vi "PrepareHWI.vi"(8 "error in (no error)":errorcluster, 9 "Master Device in":refnum<class "Master Device.lvclass">, 10 "Current Variables":T1[](array[typedef]), 11 "Arduino in":refnum<class "Arduino.lvclass">) -> (0 "error out":errorcluster, 2 "Master Device out":refnum<class "Master Device.lvclass">, 3 "Arduino out":refnum<class "Arduino.lvclass">)   [LabVIEW 2013, in "Arduino.lvclass"]
doc: "Prepare HWI will parse string table values to generate a hardware image for each device. Both variables and user functions can be pre-registered! This makes setting variables optional."
uses:
  Arduino.lvclass
  TypeDefs/Active procedure variables.ctl
  Master Device/Master Device.lvclass
  Arduino.lvclass/Arduino.ctl
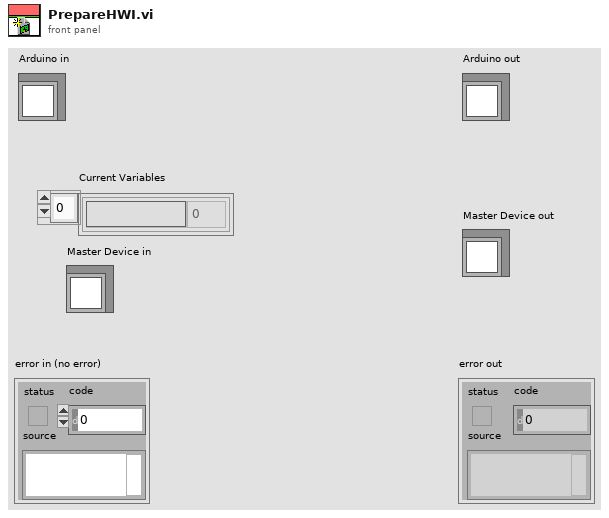
[diagram p1: front panel]
types:
  T1 = typedef "Active procedure variables.ctl" = cluster{"Procedure variable":string, "Value":dbl}
  T2 = cluster{"Short Command":string, "ParamTotal":dbl, "Params":dbl[]}[][]
  T3 = cluster{"Short Command":string, "ParamTotal":dbl, "Params":dbl[]}[]
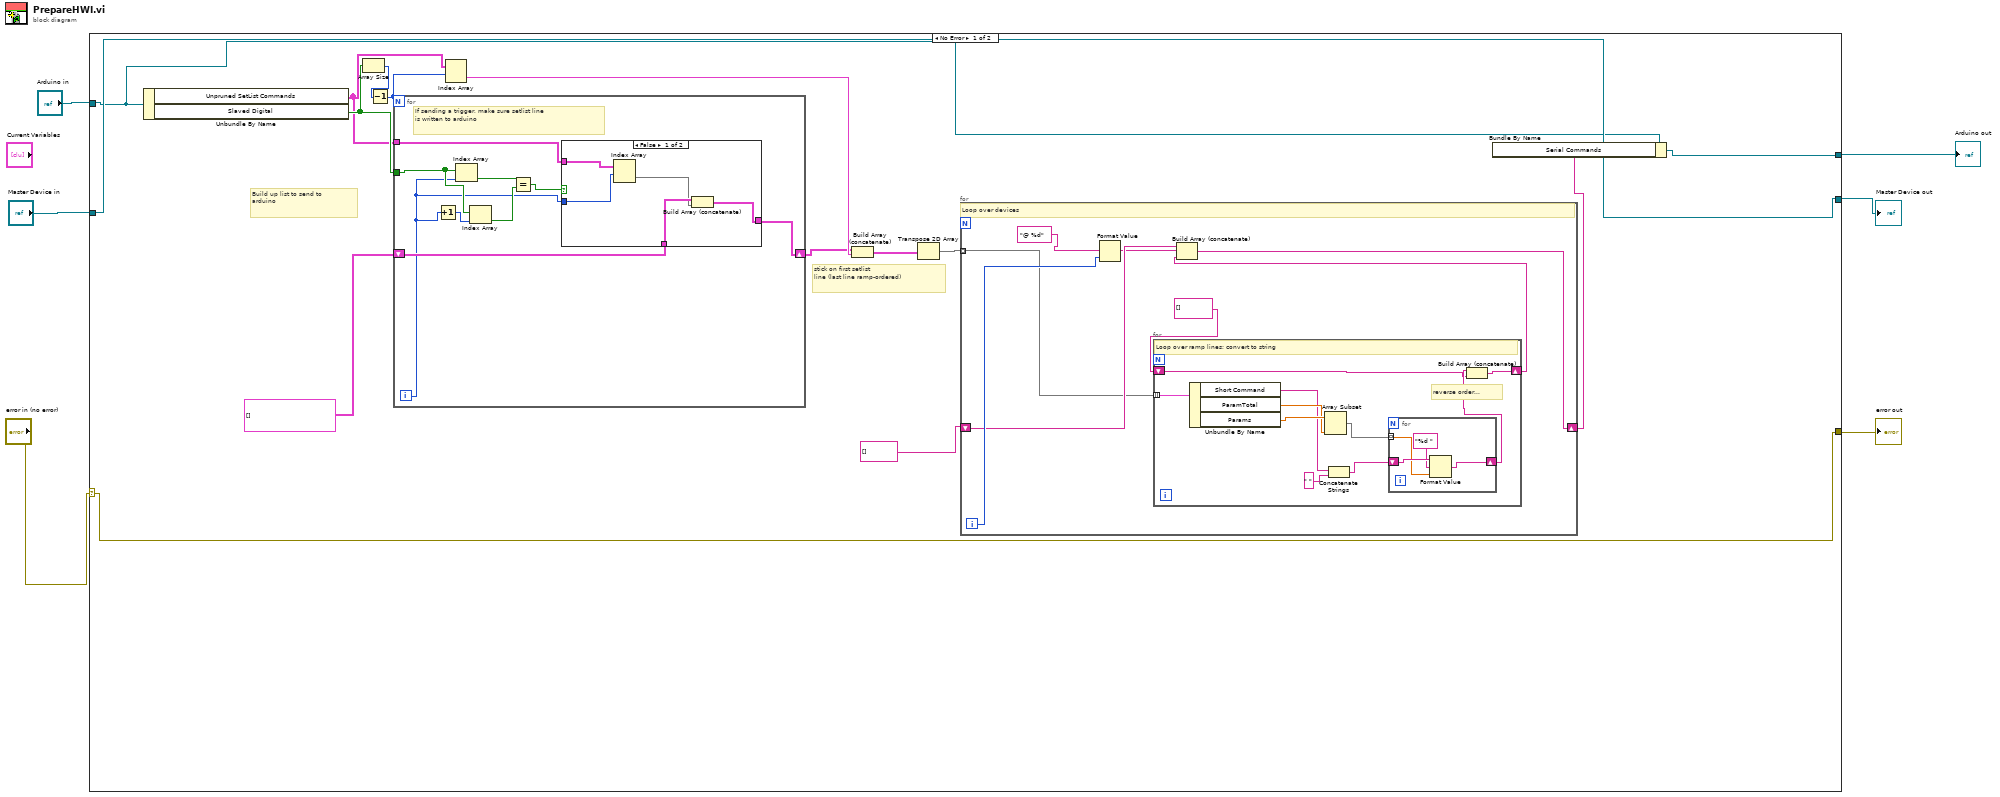
[diagram p0: block diagram]
diagram:
  n1 = case shown="No Error" "error in (no error)" {
    selector: "error in (no error)" -> [w13 w61]
    tunnel: [w13 w61] -> w6
    tunnel: [w19 w60] -> w5
    tunnel: "Master Device in" -> [w19 w60]
    tunnel: [w14 w59] -> w3
    tunnel: "Arduino in" -> [w16 w59]
    frame No Error {
      # "stick on first setlist\nline (last line ramp-ordered)"
      # "Build up list to send to\narduino"
      n2 = Unbundle By Name(w16) -> ("Unpruned SetList Commands"=w11:T2, "Slaved Digital"=w20:bool[])
      n3 = Array Size(array=w20) -> (size(s)=w12:i32)
      n4 = Decrement(x=w12) -> (x-1=w10:i32)
      n5 = for {
        N: w10 -> [_]
        tunnel: w11 -> [w45]
        tunnel: w20 -> [w51]
        shift-right: [w47] -> w8
        shift-left: T2 [] ("Unpruned SetList Commands") -> [w46]
        i -> [w44]
        # "If sending a trigger, make sure setlist line\nis written to arduino"
        n6 = Increment(x=w44) -> (x+1=w52:i32)
        n7 = Index Array(array=w51, index=w44) -> (element=w50:bool)
        n8 = Index Array(array=w51, index=w52) -> (element=w49:bool)
        n9 = Equal?(x=w50, y=w49) -> (x = y?=w48:bool)
        n10 = case shown="False" w48 {
          tunnel: [w56 w58] -> w47
          tunnel: w46 -> [w57 w58]
          tunnel: w45 -> [w55 _]
          tunnel: w44 -> [w54 _]
          frame False {
            n11 = Index Array(array=w55, index (row)=w54) -> (element=w53:T3)  [unwired: 1 in]
            n12 = Build Array (concatenate)(w57, w53) -> (w56:T2)
          }
          frame True {
          }
        }
      }
      n13 = Index Array(array=w11, index (row)=w10) -> (element=w9:T3)  [unwired: 1 in]
      n14 = Build Array (concatenate)(w8, w9) -> (w7:T2)
      n15 = Transpose 2D Array(2D array=w7) -> (transposed array=w18:T2)
      n16 = for {
        tunnel: w18 -> [w25] mode=indexing
        shift-right: [w22] -> w15
        shift-left: string[] [] -> [w27]
        i -> [w28]
        # "Loop over devices"
        n17 = Format Value(format string="@ %d", value (0)=w28) -> (output string=w26:string)  [unwired: 1 in]
        n18 = for {
          tunnel: w25 -> [w39] mode=indexing
          shift-right: [w34] -> w23
          shift-left: string[] [] ("appended array") -> [w30]
          # "reverse order..."
          # "Loop over ramp lines; convert to string"
          n19 = Unbundle By Name(w39) -> ("Short Command"=w36:string, "ParamTotal"=w37:dbl, "Params"=w38:dbl[])
          n20 = Array Subset(array=w38, length=w37) -> (w33:dbl[])  [unwired: 1 in]
          n21 = Concatenate Strings(w36, " ") -> (w32:string)
          n22 = for {
            tunnel: w33 -> [w41] mode=indexing
            shift-right: [w40] -> w31
            shift-left: w32 -> [w43]
            n23 = Format Value(string ("")=w43, format string="%d ", value (0)=w41) -> (output string=w40:string)
          }
          n24 = Build Array (concatenate)(w31, w30) -> (w34:string[])
        }
        n25 = Build Array (concatenate)(w27, w26, w23) -> (w22:string[])
      }
      n26 = Bundle By Name(cluster=w16, "Serial Commands"=w15) -> (w14:refnum<class "Arduino.lvclass">)
    }
    frame Error {
    }
  }
  "error out" <- w6
  "Arduino out" <- w3
  "Master Device out" <- w5
